vi "FXP18 to IQ.vi"(2 "I in":fxp<+/-,18,1>[](array[numeric])=[0.0, 0.0, 0.0, 0.0], 3 "Q in":fxp<+/-,18,1>[](array[numeric])=[0.0, 0.0, 0.0, 0.0]) -> (7 "data out":T1[](array[typedef]))   [LabVIEW 2018, in "GettingStarted_5774_FPGA.lvlib"]
uses:
  <instrlib>/_niInstr/DSP/v1/Shared/Public/IQ Data.ctl
  GettingStarted_5774_FPGA.lvlib
  <instrlib>/_niInstr/DSP/v1/Shared/niInstr DSP v1 Shared.lvlib
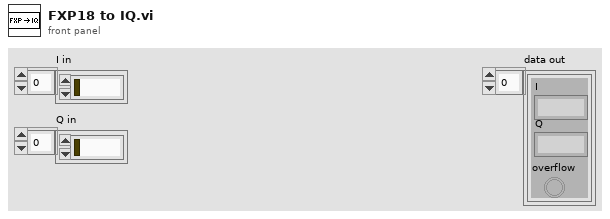
[diagram p1: front panel]
types:
  T1 = typedef "niInstr DSP v1 Shared.lvlib/IQ Data.ctl" = cluster{"I":fxp<+/-,18,1>, "Q":fxp<+/-,18,1>, "overflow":bool}
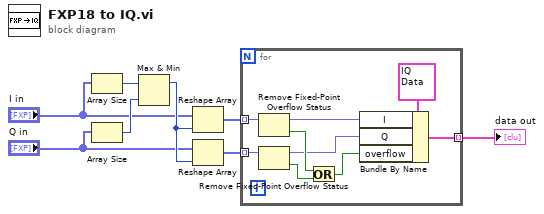
[diagram p0: block diagram]
diagram:
  n1 = Array Size(array="I in") -> (size(s)=w8:i32)
  n2 = Array Size(array="Q in") -> (size(s)=w7:i32)
  n3 = Max & Min(x=w8, y=w7) -> (max(x,y)=w6:i32)  [unwired: 1 out]
  n4 = Reshape Array("I in", w6) -> (w5:fxp<+/-,18,1>[])
  n5 = Reshape Array("Q in", w6) -> (w4:fxp<+/-,18,1>[])
  n6 = for {
    tunnel: w5 -> [w17] mode=indexing
    tunnel: w4 -> [w16] mode=indexing
    tunnel: [w11] -> w3 mode=indexing
    n7 = Remove Fixed-Point Overflow Status(3:w17) -> (0:w13:bool, 1:w10:fxp<+/-,18,1>)
    n8 = Remove Fixed-Point Overflow Status(3:w16) -> (0:w14:bool, 1:w9:fxp<+/-,18,1>)
    n9 = Or(x=w13, y=w14) -> (x .or. y?=w12:bool)
    n10 = Bundle By Name(cluster=T1 {"I"=0.0, "Q"=0.0, "overflow"=FALSE} ("IQ"), "I"=w10, "Q"=w9, "overflow"=w12) -> (w11:T1)
  }
  "data out" <- w3
